vi "Retrieve Bus B Raw Log.vi"(5 "Component ID":u8, 7 "FPGA Interface":refnum<class "FPGA Interface.lvclass">, 8 "error in (no error)":errorcluster, 11 "Bus Monitor in":refnum<class "Bus Monitor.lvclass">) -> (0 "error out":errorcluster, 2 "Bus A Raw Log":u16[](array[numeric]) format="%.0x", 3 "Bus Monitor out":refnum<class "Bus Monitor.lvclass">)   [LabVIEW 2016, in "BCI-1553 API.lvlib" / "Bus Monitor.lvclass"]
doc: "Retrieves and loosely organizes the contents of the Bus A monitor buffer."
uses:
  Bus Monitor.lvclass
  TypeDefs/Bus Monitor Read Config.ctl
  Dependencies/FPGA Interface/FPGA Interface.lvclass
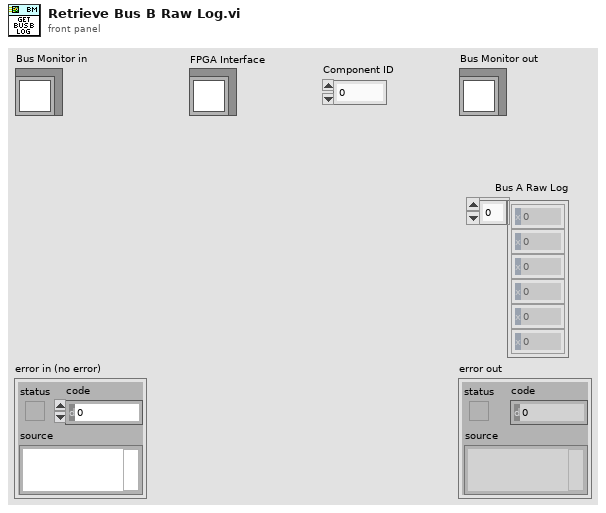
[diagram p1: front panel]
types:
  T1 = typedef "BCI-1553 API.lvlib/Bus Monitor.lvclass/Bus Monitor Read Config.ctl" = cluster{"cmdRecordStart":u16, "cmdRecordLength":u16, "dataRecordStart":u16, "dataRecordEnd":u16}
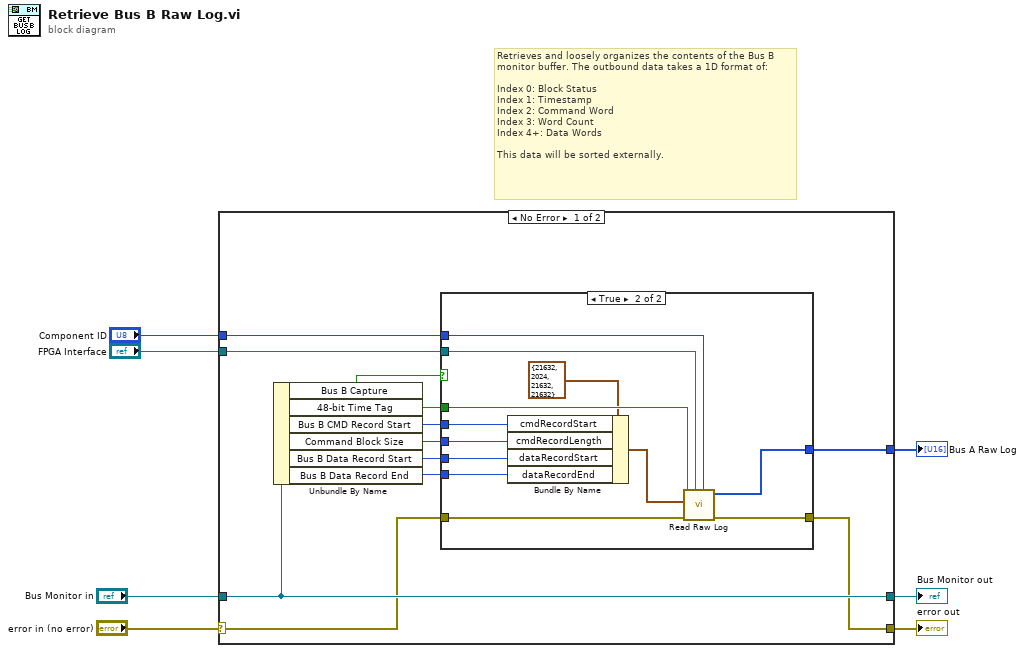
[diagram p0: block diagram]
diagram:
  # "Retrieves and loosely organizes the contents of the Bus B\nmonitor buffer. The outbound data takes a 1D format of:\n\nIndex 0: Block Status\nIndex 1: Timestamp\nIndex 2: Command Word\nIndex 3: Word Count\nIndex 4+: Data Words\n\nThis data will be sorted externally."
  n1 = case shown="No Error" "error in (no error)" {
    selector: "error in (no error)" -> [w18 w33]
    tunnel: [w10 w33] -> w6
    tunnel: [w19 w32] -> w4
    tunnel: "Bus Monitor in" -> [w19 w32]
    tunnel: [w11 _] -> w3
    tunnel: "FPGA Interface" -> [w13 _]
    tunnel: "Component ID" -> [w12 _]
    frame No Error {
      n2 = Unbundle By Name(w19) -> ("Bus B Capture"=w14:bool, "48-bit Time Tag"=w15:bool, "Bus B CMD Record Start"=w16:u16, "Command Block Size"=w17:u16, "Bus B Data Record Start"=w9:u16, "Bus B Data Record End"=w8:u16)
      n3 = case shown="True" w14 {
        tunnel: [_ w27] -> w11
        tunnel: w13 -> [_ w29]
        tunnel: w12 -> [_ w28]
        tunnel: [_ w26] -> w10
        tunnel: w17 -> [_ w23]
        tunnel: w16 -> [_ w24]
        tunnel: w15 -> [_ w30]
        tunnel: w18 -> [_ w31]
        tunnel: w9 -> [_ w22]
        tunnel: w8 -> [_ w21]
        frame False {
        }
        frame True {
          n4 = Bundle By Name(cluster=T1 {"cmdRecordStart"=21632, "cmdRecordLength"=2024, "dataRecordStart"=21632, "dataRecordEnd"=21632} ("bmReadConfig"), "cmdRecordStart"=w24, "cmdRecordLength"=w23, "dataRecordStart"=w22, "dataRecordEnd"=w21) -> (w20:T1)
          n5 = call "Read Raw Log.vi"("Component ID"=w28, "FPGA Interface"=w29, "error in (no error)"=w31, "bmReadConfig"=w20, "48-bit Timetag?"=w30) -> ("error out"=w26:errorcluster, "Raw Log"=w27:u16[])  [unwired: 5 in]
        }
      }
    }
    frame Error {
    }
  }
  "error out" <- w6
  "Bus Monitor out" <- w4
  "Bus A Raw Log" <- w3
